vi "New SSL Client Socket.vi"(6 "Verify hostname? (T)":bool=TRUE, 8 "error in (no error)":errorcluster, 10 "Hostname / URL":string="echo.websocket.org:443", 11 "SSL Client Ctx":refnum<class "SSL Client Context.lvclass">) -> (0 "error out":errorcluster, 3 "SSL Client Skt out":refnum<class "SSL Client Socket.lvclass">)   [LabVIEW 2013, in "OpenSSL Socket.lvlib" / "SSL Client Socket.lvclass"]
doc: "Creates a new SSL Client Socket and connects to the server."
uses:
  SSL Client Socket.lvclass
  SSL Client Context/SSL Client Context.lvclass
  SSL Client Socket.lvclass/SSL Client Socket.ctl
  Write Server Hostname.vi
  Write Verify hostname.vi
  <vilib>/MediaMongrels Ltd/WebSockets/WebSockets/WebSocket Client/WebSocket Client.lvclass
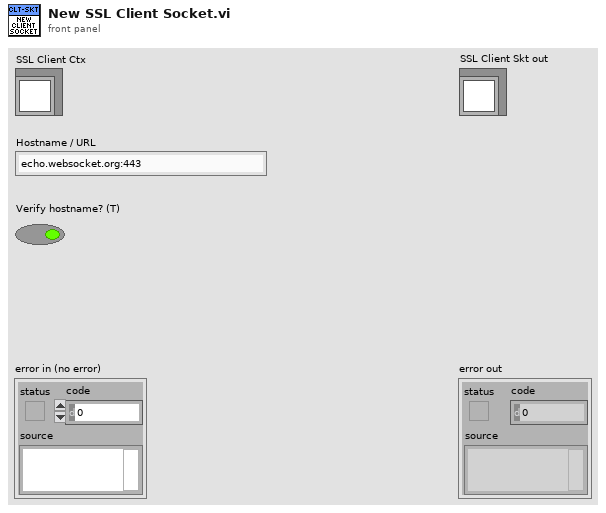
[diagram p1: front panel]
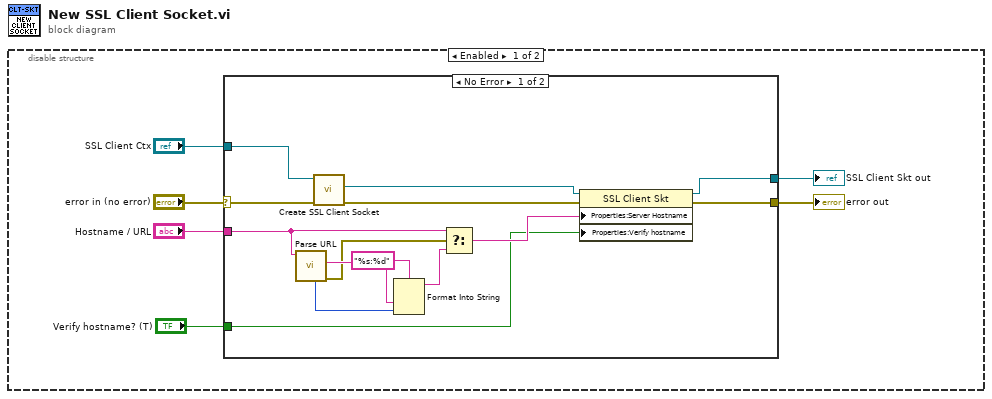
[diagram p0: block diagram]
diagram:
  n1 = disable-structure shown="Enabled" {
    frame Enabled {
      n2 = case shown="No Error" "error in (no error)" {
        selector: "error in (no error)" -> [w14 w21]
        tunnel: [w10 w21] -> w5
        tunnel: "SSL Client Ctx" -> [w13 _]
        tunnel: "Hostname / URL" -> [w15 _]
        tunnel: [w11 _] -> w2
        tunnel: "Verify hostname? (T)" -> [w8 _]
        frame No Error {
          n3 = call <vilib>:"Parse URL.vi"("WebSocket URL"=w15) -> ("error out"=w17:errorcluster, "host"=w20:string, "port"=w19:u16)  [unwired: 6 in, 2 out]
          n4 = call "Create SSL Client Socket.vi"("error in (no error)"=w14, "SSL Client Ctx in"=w13) -> ("error out"=w12:errorcluster, "SSL Client Socket"=w7:refnum<class "SSL Client Socket.lvclass">)  [unwired: 7 in, 1 out]
          n5 = Format Into String(format string="%s:%d", w20, w19) -> (resulting string=w16:string)  [unwired: 2 in, 1 out]
          n6 = Select(t=w15, s=w17, f=w16) -> (s? t:f=w9:string)
          n7 = property class="SSL Client Skt"(reference=w7, error in=w12, "Properties:Server Hostname"=w9, "Properties:Verify hostname"=w8) -> (reference out=w11:refnum<class "SSL Client Socket.lvclass">, error out=w10:errorcluster)
        }
        frame Error {
        }
      }
      "error out" <- w5
      "SSL Client Skt out" <- w2
    }
    frame Disabled {
    }
  }
